vi "parse frame.vi"(8 "error in (no error)":errorcluster, 11 "<f> string":string) -> (0 "error out":errorcluster, 3 "frame data":T1)   [LabVIEW 2018, in "Data Parser.lvclass"]
uses:
  Data Parser.lvclass
  frame data.ctl
  frame title.ctl
  frame basic data.ctl
  frame o data.ctl
  frame bp data.ctl
  frame c data.ctl
  frame w data.ctl
  frame i data.ctl
  frame b data.ctl
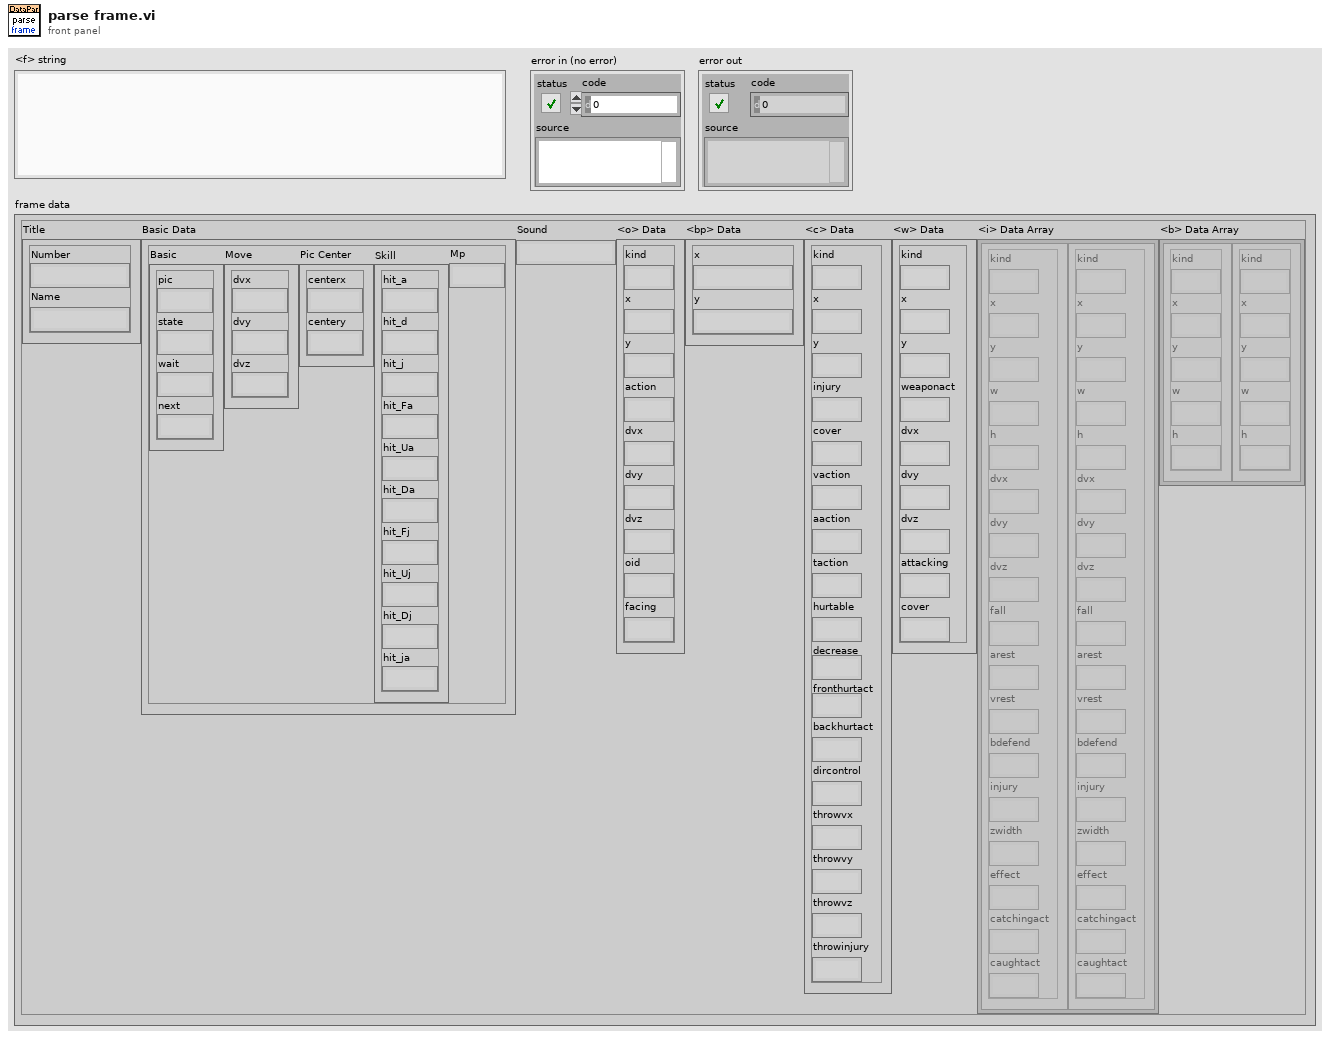
[diagram p1: front panel]
types:
  T1 = typedef "Data Parser.lvclass/frame data.ctl" = cluster{"Title":T2, "Basic Data":T3, "Sound":string, "<o> Data":T4, "<bp> Data":T5, "<c> Data":T6, "<w> Data":T7, "<i> Data Array":T8[], "<b> Data Array":T9[]}
  T2 = typedef "Data Parser.lvclass/frame title.ctl" = cluster{"Number":string, "Name":string}
  T3 = typedef "Data Parser.lvclass/frame basic data.ctl" = cluster{"Basic":cluster{"pic":string, "state":string, "wait":string, "next":string}, "Move":cluster{"dvx":string, "dvy":string, "dvz":string}, "Pic Center":cluster{"centerx":string, "centery":string}, "Skill":cluster{"hit_a":string, "hit_d":string, "hit_j":string, "hit_Fa":string, "hit_Ua":string, "hit_Da":string, "hit_Fj":string, "hit_Uj":string, "hit_Dj":string, "hit_ja":string}, "Mp":string}
  T4 = typedef "Data Parser.lvclass/frame o data.ctl" = cluster{"kind":string, "x":string, "y":string, "action":string, "dvx":string, "dvy":string, "dvz":string, "oid":string, "facing":string}
  T5 = typedef "Data Parser.lvclass/frame bp data.ctl" = cluster{"x":string, "y":string}
  T6 = typedef "Data Parser.lvclass/frame c data.ctl" = cluster{"kind":string, "x":string, "y":string, "injury":string, "cover":string, "vaction":string, "aaction":string, "taction":string, "hurtable":string, "decrease":string, "fronthurtact":string, "backhurtact":string, "dircontrol":string, "throwvx":string, "throwvy":string, "throwvz":string, "throwinjury":string}
  T7 = typedef "Data Parser.lvclass/frame w data.ctl" = cluster{"kind":string, "x":string, "y":string, "weaponact":string, "dvx":string, "dvy":string, "dvz":string, "attacking":string, "cover":string}
  T8 = typedef "Data Parser.lvclass/frame i data.ctl" = cluster{"kind":string, "x":string, "y":string, "w":string, "h":string, "dvx":string, "dvy":string, "dvz":string, "fall":string, "arest":string, "vrest":string, "bdefend":string, "injury":string, "zwidth":string, "effect":string, "catchingact":string, "caughtact":string}
  T9 = typedef "Data Parser.lvclass/frame b data.ctl" = cluster{"kind":string, "x":string, "y":string, "w":string, "h":string}
  T10 = cluster{"frame info":string, "basic":string, "sound":string, "<bp> body point":string, "<w> weapon":string, "<b> body array":string[], "<i> injury array":string[], "<o> object":string, "<c> catch":string}
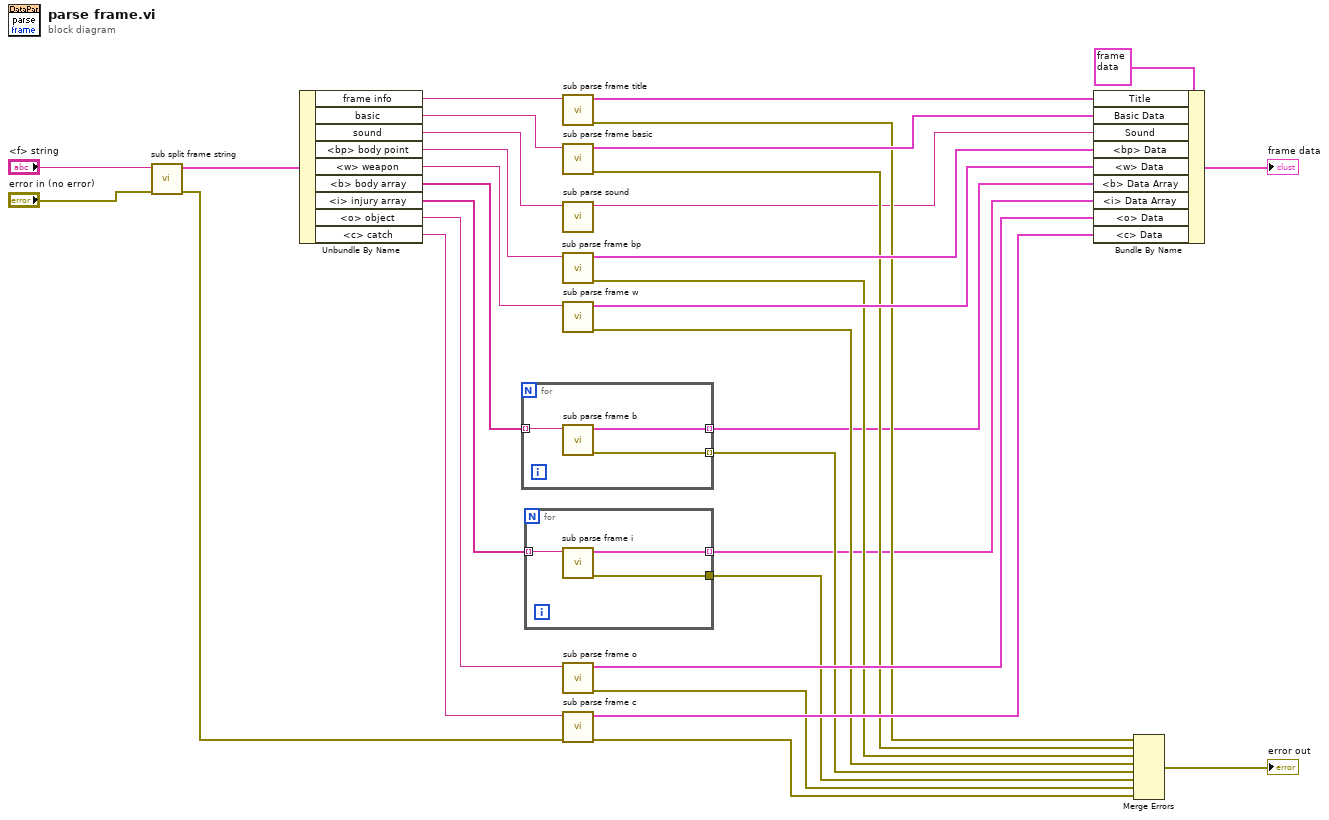
[diagram p0: block diagram]
diagram:
  n1 = call "sub split frame string.vi"("error in (no error)"="error in (no error)", "frame string"="<f> string") -> ("error out"=w18:errorcluster, "split string"=w33:T10)  [unwired: 8 in]
  n2 = Unbundle By Name(w33) -> ("frame info"=w32:string, "basic"=w31:string, "sound"=w2:string, "<bp> body point"=w30:string, "<w> weapon"=w28:string, "<b> body array"=w7:string[], "<i> injury array"=w27:string[], "<o> object"=w26:string, "<c> catch"=w19:string)
  n3 = for {
    tunnel: [w36] -> w12 mode=indexing
    tunnel: w7 -> [w35] mode=indexing
    tunnel: [w34] -> w6 mode=indexing
    n4 = call "sub parse frame b.vi"("<b> String"=w35) -> ("error out"=w36:errorcluster, "<b> data"=w34:T9)  [unwired: 9 in]
  }
  n5 = for {
    tunnel: w27 -> [w39] mode=indexing
    tunnel: [w38] -> w11
    tunnel: [w37] -> w3 mode=indexing
    n6 = call "sub parse frame i.vi"("<i> String"=w39) -> ("error out"=w38:errorcluster, "<i> data"=w37:T8)  [unwired: 9 in]
  }
  n7 = call "sub parse frame title.vi"("String"=w32) -> ("error out"=w16:errorcluster, "frame title"=w24:T2)  [unwired: 9 in]
  n8 = call "sub parse frame basic.vi"("String"=w31) -> ("error out"=w15:errorcluster, "frame basic data"=w23:T3)  [unwired: 9 in]
  n9 = call "sub parse sound.vi"("sound string"=w2) -> ("sound"=w1:string)  [unwired: 9 in, 1 out]
  n10 = call "sub parse frame bp.vi"("<bp> String"=w30) -> ("error out"=w14:errorcluster, "bp data"=w22:T5)  [unwired: 9 in]
  n11 = call "sub parse frame w.vi"("<w> String"=w28) -> ("error out"=w13:errorcluster, "w data"=w21:T7)  [unwired: 9 in]
  n12 = call "sub parse frame o.vi"("<o> String"=w26) -> ("error out"=w10:errorcluster, "<o> data"=w20:T4)  [unwired: 9 in]
  n13 = call "sub parse frame c.vi"("error in (no error)"=w18, "<c> String"=w19) -> ("error out"=w9:errorcluster, "<c> data"=w17:T6)  [unwired: 8 in]
  n14 = Bundle By Name(cluster=T1 {"Title"={"Number"="60", "Name"="-"}, "Basic Data"={"Basic"={"pic"="10", "state"="3", "wait"="3", "next"="61"}, "Move"={"dvx"="", "dvy"="", "dvz"=""}, "Pic Center"={"centerx"="45", "centery"=""}, "Skill"={"hit_a"="", "hit_d"="", "hit_j"="", "hit_Fa"="", "hit_Ua"="", "hit_Da"="", "hit_Fj"="", "hit_Uj"="", "hit_Dj"="", "hit_ja"=""}, "Mp"=""}, "Sound"="", "<o> Data"={"kind"="", "x"="", "y"="", "action"="", "dvx"="", "dvy"="", "dvz"="", "oid"="", "facing"=""}, "<bp> Data"={"x"="48.75061461791846", "y"="38.42940829813039"}, "<c> Data"={"kind"="", "x"="", "y"="", "injury"="", "cover"="", "vaction"="", "aaction"="", "taction"="", "hurtable"="", "decrease"="", "fronthurtact"="", "backhurtact"="", "dircontrol"="", "throwvx"="", "throwvy"="", "throwvz"="", "throwinjury"=""}, "<w> Data"={"kind"="", "x"="", "y"="", "weaponact"="", "dvx"="", "dvy"="", "dvz"="", "attacking"="", "cover"=""}, "<i> Data Array"=[], "<b> Data Array"=[{"kind"="0", "x"="28", "y"="20", "w"="31", "h"="63"}]} ("frame data 2"), "Title"=w24, "Basic Data"=w23, "Sound"=w1, "<bp> Data"=w22, "<w> Data"=w21, "<b> Data Array"=w6, "<i> Data Array"=w3, "<o> Data"=w20, "<c> Data"=w17) -> (→"frame data":T1)
  n15 = Merge Errors(w16, w15, w14, w13, w12, w11, w10, w9) -> (→"error out":errorcluster)
